vi "get name.vi"(8 "error in (no error)":errorcluster caption="Fehler (Eingang, kein Fehler)", 11 "Segment (Eingang)":refnum<class "Test.lvclass">) -> (0 "error out":errorcluster caption="Fehler (Ausgang)", 2 "name":string, 3 "Segment (Ausgang)":refnum<class "Test.lvclass">)   [LabVIEW 2013, in "DatenKlassen.lvlib" / "Test.lvclass"]
uses:
  Test.lvclass
  Test.lvclass/Test.ctl
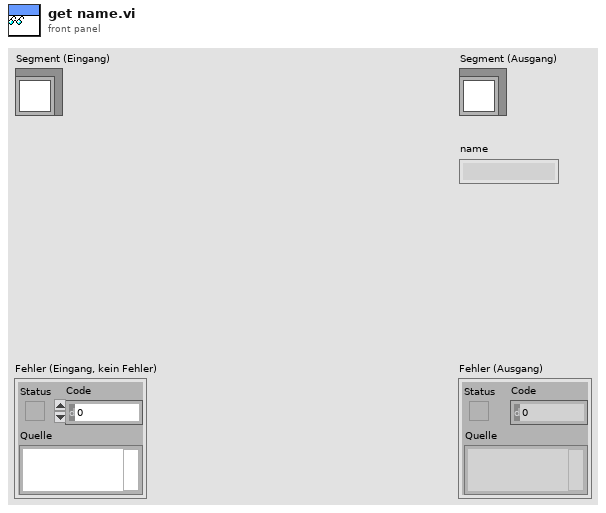
[diagram p1: front panel]
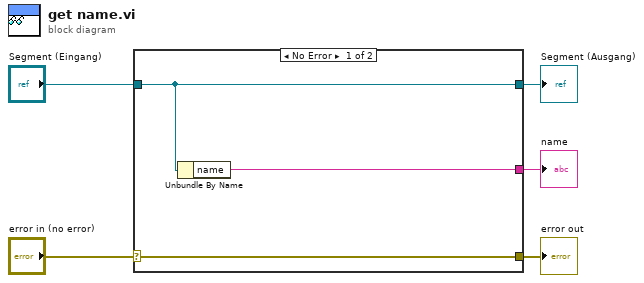
[diagram p0: block diagram]
diagram:
  n1 = case shown="No Error" "error in (no error)" {
    selector: "error in (no error)" -> [w8 w9]
    tunnel: [w8 w9] -> w4
    tunnel: [w7 w10] -> w2
    tunnel: "Segment (Eingang)" -> [w7 w10]
    tunnel: [w6 _] -> w1
    frame No Error {
      n2 = Unbundle By Name(w7) -> ("name"=w6:string)
    }
    frame Error {
    }
  }
  "error out" <- w4
  "Segment (Ausgang)" <- w2
  "name" <- w1
